vi "XYZStage-Set max speed command.vi"(8 "Error In":errorcluster, 9 "XYZ Stage data":T1={"Command"=enum."Initialize", "Channel"="Z", "X"=0.0, "Y"=0.0, "Z"=0.0, "Speed"=0, "Zero"=FALSE, "Use acknowledgement?"=TRUE} {"Speed" format="Speed= %.0f"; "Z" format="Z= %#_g"; "Y" format="Y= %#_g"; "X" format="X= %#_g"}, 11 "XYZ Stage config":T4={"COM port"="COM7", "XY stage available"=FALSE}) -> (0 "Error Out":errorcluster)   [LabVIEW 2013]
uses:
  Typedefs/XY Stage config cluster.ctl
  Typedefs/XYZ stage data.ctl
  Typedefs/XYZ stage states.ctl
  Typedefs/XYZ channel ring.ctl
panel:
  out "read string":string
  out "Set max speed command string":string
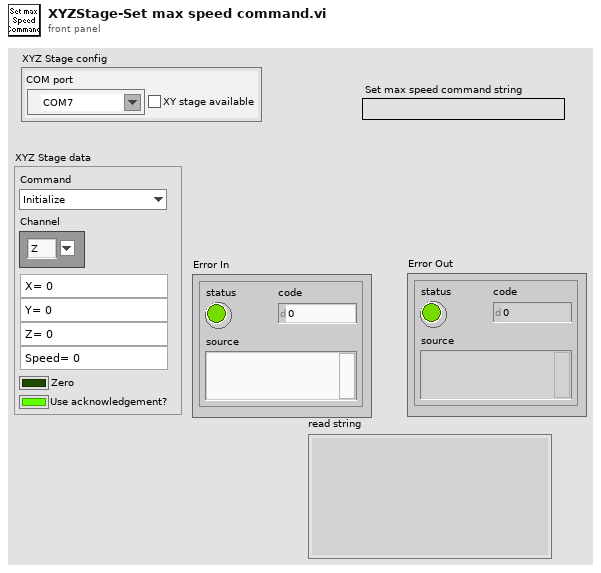
[diagram p1: front panel]
types:
  T1 = typedef "XYZ stage data.ctl" = cluster{"Command":T2, "Channel":T3, "X":sgl, "Y":sgl, "Z":sgl, "Speed":i32, "Zero":bool, "Use acknowledgement?":bool}
  T2 = typedef "XYZ stage states.ctl" = enum16{"Dequeue", "Initialize", "Read Position", "Read Speed Setting", "Move", "Set Max Speed", "Reset Axis", "Stop all movement"}
  T3 = typedef "XYZ channel ring.ctl" = string
  T4 = typedef "XY Stage config cluster.ctl" = cluster{"COM port":refnum<visa-resource-name>, "XY stage available":bool}
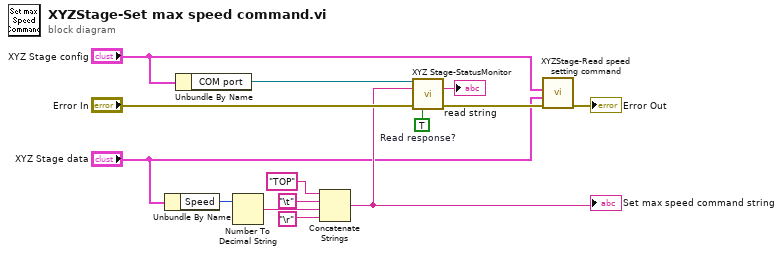
[diagram p0: block diagram]
diagram:
  w13 = TRUE  # Read response?
  n1 = Unbundle By Name("XYZ Stage data") -> ("Speed"=w8:i32)
  n2 = Unbundle By Name("XYZ Stage config") -> ("COM port"=w7:refnum<visa-resource-name>)
  n3 = Number To Decimal String(number=w8) -> (decimal integer string=w12:string)  [unwired: 1 in]
  n4 = Concatenate Strings("TOP" ("decimal integer string"), "\t" ("Tab Constant"), w12, "\r" ("Carriage Return Constant")) -> (w6:string)
  "Set max speed command string" <- w6
  n5 = call "XYZ Stage-StatusMonitor.vi"("VISA resource name"=w7, "string to write"=w6, "Error In"="Error In", "Read response? (T)"=w13) -> ("read string"=→"read string":string, "Error Out"=w5:errorcluster)  [unwired: 7 in, 3 out]
  n6 = call "XYZStage-Read speed setting command.vi"("error in (no error)"=w5, "XYZ Stage data to queue"="XYZ Stage data", "XY Stage config cluster"="XYZ Stage config") -> ("error out"=→"Error Out":errorcluster)  [unwired: 8 in]
